vi "setAcqFormat.vi"(8 "error in (no error)":errorcluster, 9 "acquisition format":T1, 10 "number of ROIs":i32, 11 "CCD in":refnum<class "CCD.lvclass">) -> (0 "error out":errorcluster, 1 "ID":i32, 2 "results-JSON string":string, 3 "CCD out":refnum<class "CCD.lvclass">)   [LabVIEW 2023, in "CCD.lvclass"]
uses:
  CCD.lvclass
  CCD.lvclass/CCD.ctl
  20f7d3bd-08ac-4524-9bed-df36c1da25a0.vi
  GenericDevice/GenericDevice.lvclass
  9c26a383-523e-4ef9-a52a-706f8f4d1e65.vi
  1afe4a3d-b8bf-4f9d-9cc3-ba347473a4dc.vi
  <vilib>/IlluminatedG/lv-web-crypto/lv-json/JSON/JSON.lvlib
  AcquisitionFormatEnum.ctl
panel:
  # "Connector Pane"
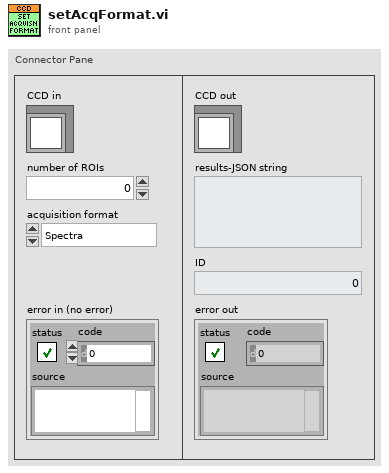
[diagram p1: front panel]
types:
  T1 = typedef "CCD.lvclass/AcquisitionFormatEnum.ctl" = enum16{"Spectra", "Image", "Crop", "Fast Kinetics"}
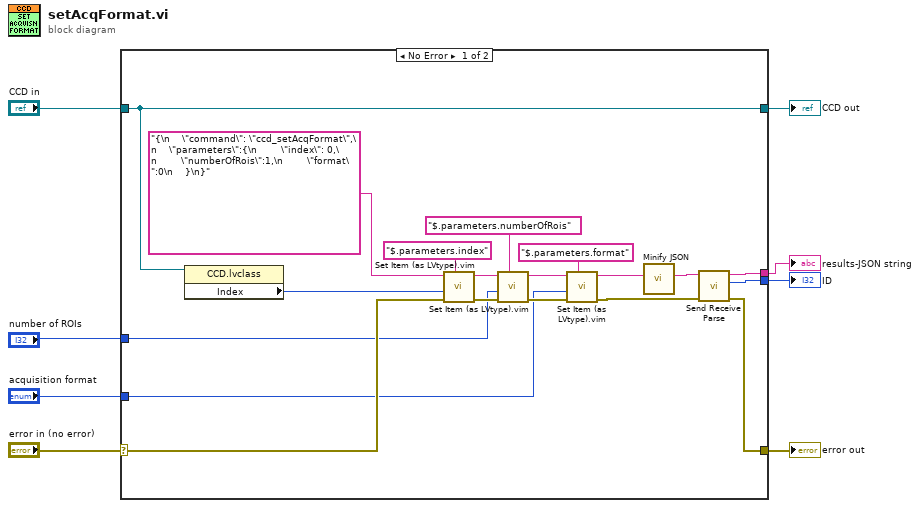
[diagram p0: block diagram]
diagram:
  n1 = case shown="No Error" "error in (no error)" {
    selector: "error in (no error)" -> [w23 w29]
    tunnel: [w13 w29] -> w7
    tunnel: [w25 w28] -> w5
    tunnel: "CCD in" -> [w25 w28]
    tunnel: "number of ROIs" -> [w15 _]
    tunnel: "acquisition format" -> [w14 _]
    tunnel: [w12 _] -> w2
    tunnel: [w11 _] -> w1
    frame No Error {
      n2 = property class="CCD.lvclass"(reference=w25) -> ("Index"=w24:i32)  [unwired: 1 in, 2 out]
      n3 = call "Set Item (as LVtype).vim"("$Path or Item Name"="$.parameters.index", "error in (no error)"=w23, "Anything"=w24, "JSON"="{\n    \"command\": \"ccd_setAcqFormat\",\n    \"parameters\":{\n        \"index\": 0,\n        \"numberOfRois\":1,\n        \"format\":0\n    }\n}") -> ("error out"=w20:errorcluster, "<JSON>"=w21:string)  [unwired: 4 in, 1 out]
      n4 = call "Set Item (as LVtype).vim"("$Path or Item Name"="$.parameters.numberOfRois", "error in (no error)"=w20, "Anything"=w15, "JSON"=w21) -> ("error out"=w18:errorcluster, "<JSON>"=w19:string)  [unwired: 4 in, 1 out]
      n5 = call "Set Item (as LVtype).vim"("$Path or Item Name"="$.parameters.format", "error in (no error)"=w18, "Anything"=w14, "JSON"=w19) -> ("error out"=w17:errorcluster, "<JSON>"=w10:string)  [unwired: 4 in, 1 out]
      n6 = call <vilib>:"Minify JSON.vi"("JSON String"=w10) -> ("Minified JSON"=w9:string)  [unwired: 10 in]
      n7 = call "Send Receive Parse.vi"("error in"=w17, "<JSON>"=w9) -> ("error out"=w13:errorcluster, "ID"=w11:i32, "results-JSON string"=w12:string)  [unwired: 7 in]
    }
    frame Error {
    }
  }
  "error out" <- w7
  "CCD out" <- w5
  "results-JSON string" <- w2
  "ID" <- w1
